vi "MRC Message Loop.vi"(8 "error in (no error)":errorcluster) -> (0 "error out":errorcluster)   [LabVIEW 2020, in "MRC Module.lvlib"]
doc: "Message loop for handling messages pertaining to the acquisition of data from the hardware."
uses:
  MRC Module.lvlib
  support/PCT FGV CMD.ctl
  Acquisition State.ctl
  MRC Configuration.ctl
  support/Message Queue/Message Cluster.ctl
  support/Message Queue/Enqueue Message (Single).vi
  support/Message Queue/Message Queue.lvlib
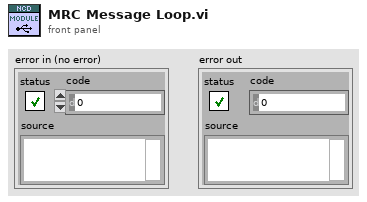
[diagram p1: front panel]
types:
  T1 = typedef "PCT FGV CMD.ctl" = enum16{"INIT", "GET", "SET"}
  T2 = typedef "Message Queue.lvlib/All Message Queues.ctl" = cluster{"UI":refnum<queue>, "Logging":refnum<queue>, "LOG":refnum<queue>, "ALARM":refnum<queue>, "Test":refnum<queue>, "Answer":refnum<queue>, "PLC":refnum<queue>, "DB":refnum<queue>, "Report":refnum<queue>, "OPC":refnum<queue>, "Procedure":refnum<queue>, "PalmSens":refnum<queue>, "SYS 7000 Reader":refnum<queue>, "SWITCH":refnum<queue>, "MOTOR":refnum<queue>, "MOTION":refnum<queue>, "HIDEN":refnum<queue>, "VALVE":refnum<queue>, "MFC":refnum<queue>, "PUMP IN":refnum<queue>, "PUMP OUT":refnum<queue>}
  T3 = typedef "PCT Data REFs.ctl" = cluster{"PLC AI Notifier":refnum<notifier>, "PS Data Queue":refnum<queue>, "BTN Queue":refnum<queue>, "PLC DI notifier":refnum<notifier>, "Timer notifier":refnum<notifier>, "DMM PS":refnum<notifier>, "DMM Gages":refnum<notifier>, "XYZ notifier":refnum<notifier>, "Test Notifier":refnum<notifier>, "Scanner notifier":refnum<notifier>, "OPC Notifier":refnum<notifier>, "HIDEN queue":refnum<queue>}
  T4 = typedef "MRC Module.lvlib/MRC Configuration.ctl" = cluster{"MFC Definition":cluster{"MFC Port":refnum<visa-resource-name>, "MFC Enable":bool, "Baud Rate":i32, "Interface type":enum32{"RS-485", "RS-232"}, "Address":i32}, "Set Point Options":cluster{"Setpoint Value":dbl, "Mass Flow EU 2":string, "Setpoint Source":string, "Valve Mode":string}, "Writer Queue":refnum<queue>, "Enable":bool, "Update Rate":u32, "MRC Chamber Enable":bool, "Selected Gas":string, "Address String":string}
  T5 = typedef "MRC Module.lvlib/Acquisition State.ctl" = enum16{"Idle", "Initialized"}
  T6 = typedef "Message Queue.lvlib/Message Cluster.ctl" = cluster{"Message":string, "Message Data":variant}
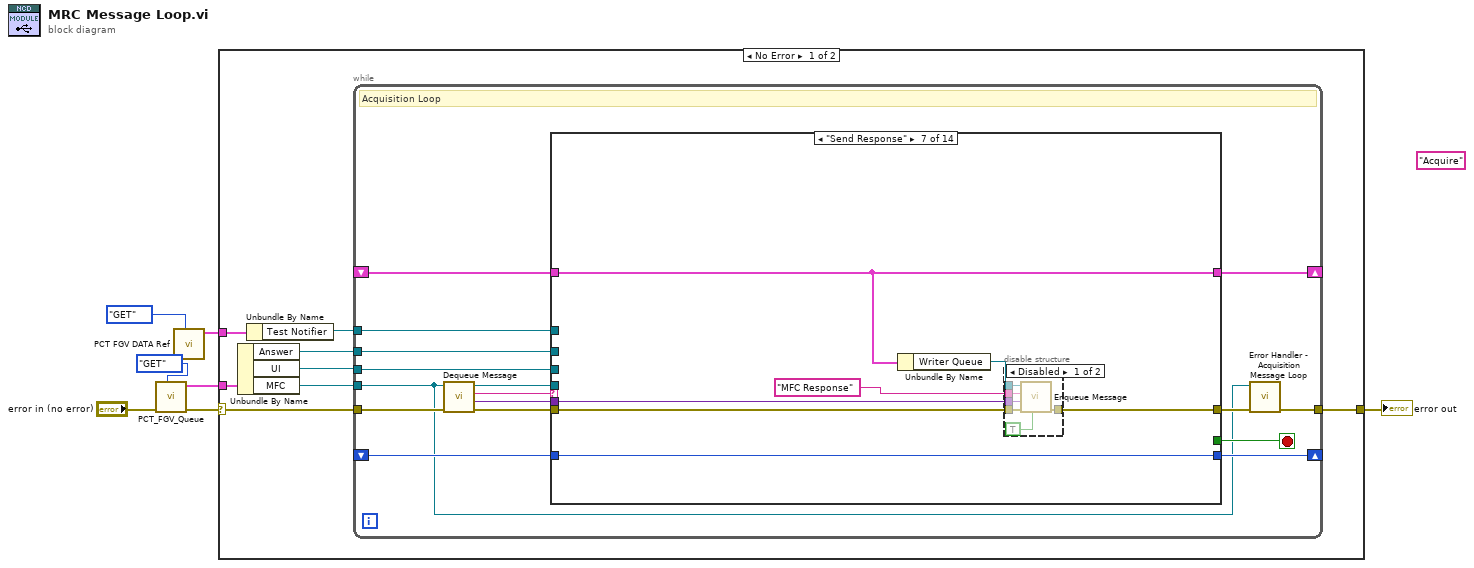
[diagram p0: block diagram]
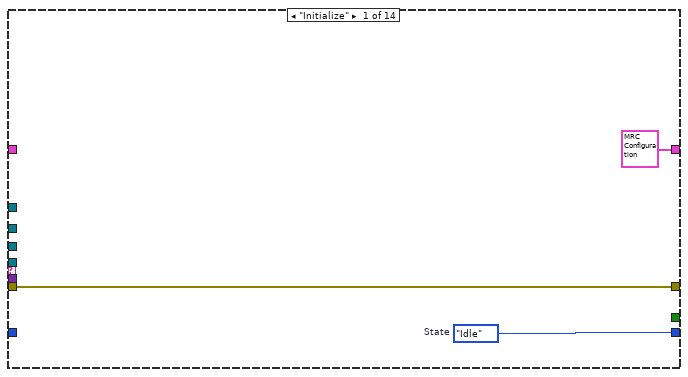
[diagram p2: hidden frame]
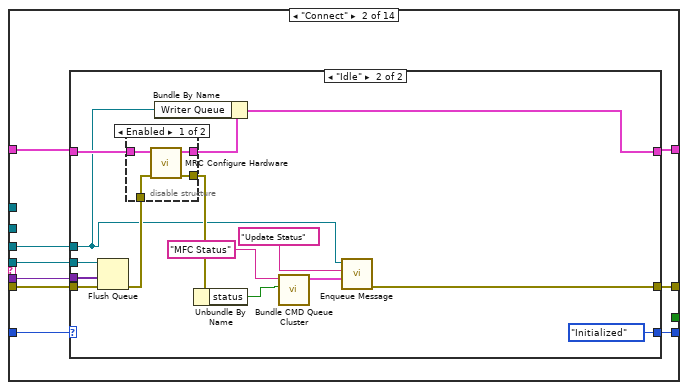
[diagram p3: hidden frame]
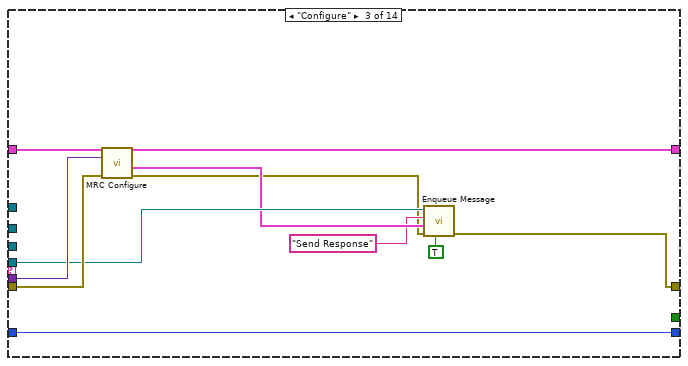
[diagram p6: hidden frame]
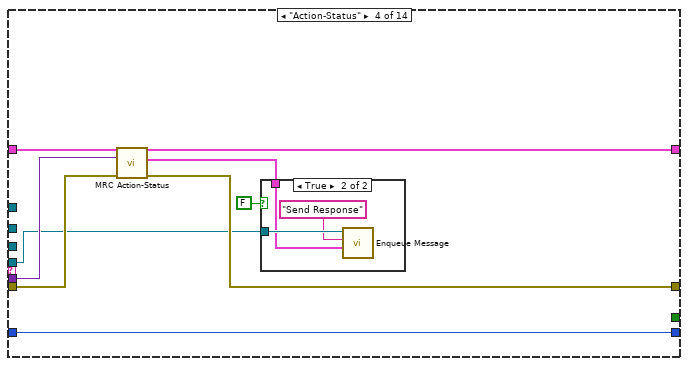
[diagram p7: hidden frame]
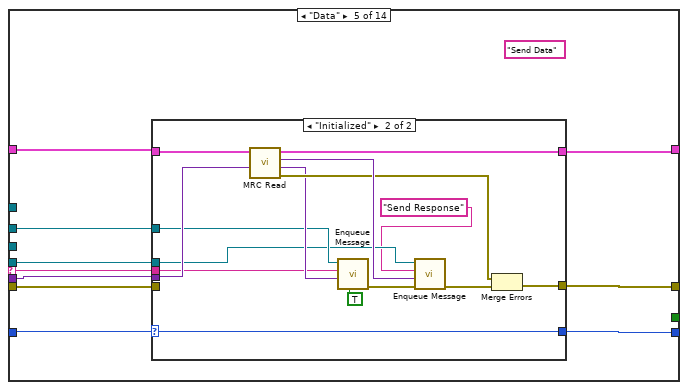
[diagram p9: hidden frame]
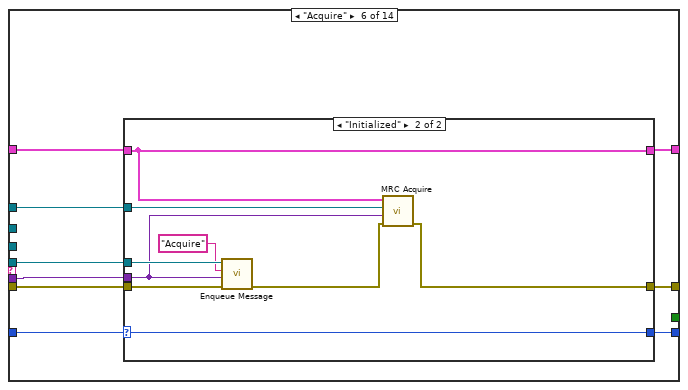
[diagram p11: hidden frame]
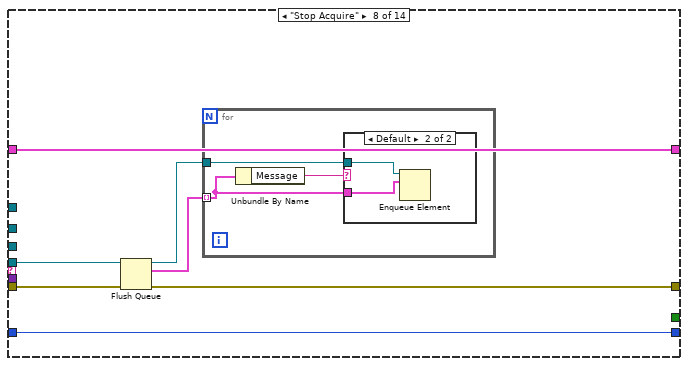
[diagram p14: hidden frame]
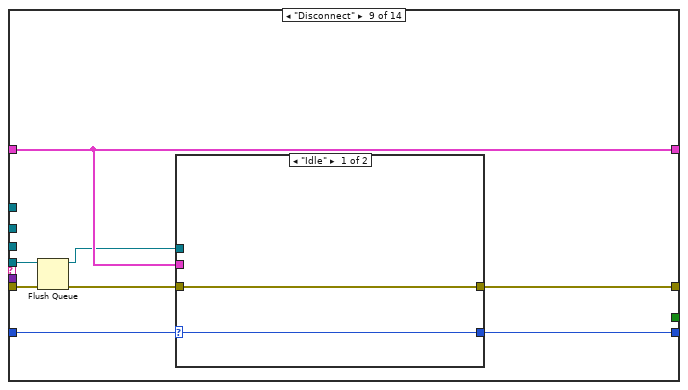
[diagram p16: hidden frame]
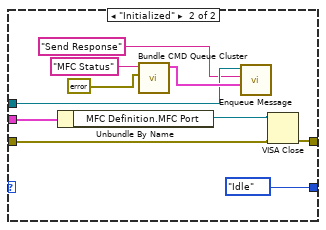
[diagram p17: hidden frame]
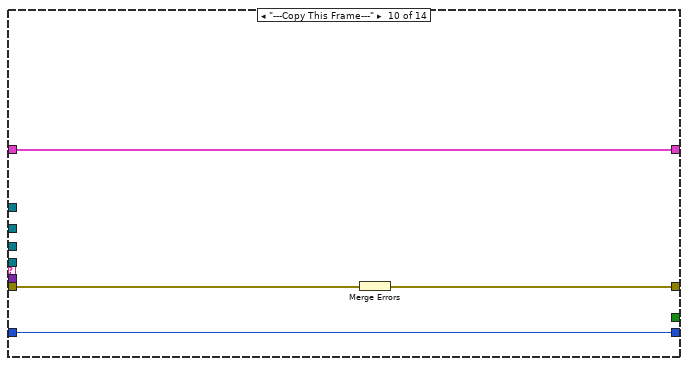
[diagram p18: hidden frame]
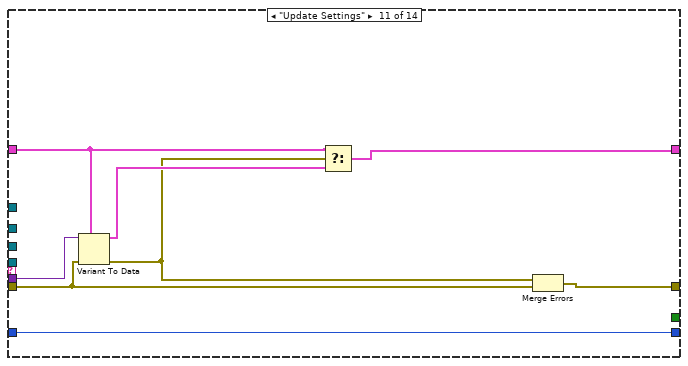
[diagram p19: hidden frame]
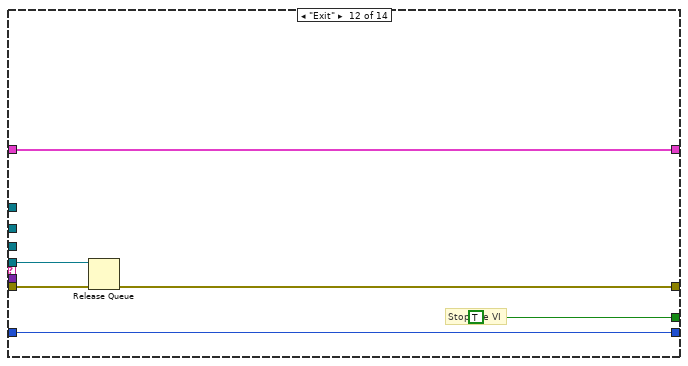
[diagram p20: hidden frame]
diagram:
  (unwired) "Acquire" ("Message")
  n1 = call "PCT_FGV_Queue.vi"("CMD"=PCT_FGV_CMD."GET", "error in (no error)"="error in (no error)") -> ("error out"=w2:errorcluster, "Message Queues out"=w1:T2)  [unwired: 8 in]
  n2 = call "PCT FGV DATA Ref.vi"("CMD"=PCT_FGV_CMD."GET") -> ("Data REF"=w5:T3)  [unwired: 9 in, 1 out]
  n3 = case shown="No Error" w2 {
    selector: w2 -> [w12 w219]
    tunnel: w1 -> [w15 _]
    tunnel: [w13 w219] -> w7
    tunnel: w5 -> [w10 _]
    frame No Error {
      n4 = Unbundle By Name(w15) -> ("Answer"=w8:refnum<queue>, "UI"=w11:refnum<queue>, "MFC"=w14:refnum<queue>)
      n5 = Unbundle By Name(w10) -> ("Test Notifier"=w9:refnum<notifier>)
      n6 = while {
        tunnel: w14 -> [w17]
        shift-right: [w30] -> _
        shift-left: _ -> [w31]
        tunnel: w11 -> [w21]
        shift-right: [w24] -> _
        shift-left: _ -> [w25]
        tunnel: w9 -> [w18]
        tunnel: w8 -> [w16]
        tunnel: w12 -> [w28]
        tunnel: [w19] -> w13
        stop <- w29 stop-if-true
        # "Acquisition Loop"
        n7 = call "Dequeue Message.vi"("error in (no error)"=w28, "Message Queue"=w17) -> ("error out"=w27:errorcluster, "Message Data"=w26:variant, "Message"=w22:string, "dup Message Queue"=w23:refnum<queue>)  [unwired: 6 in]
        n8 = case "Message Cases" shown="\"Send Response\"" w22 {
          selector: w22 -> [_ _ _ _ w91 _ _ _ _ _ _ _ _ _]
          tunnel: w23 -> [_ w40 w72 w78 w98 w125 _ w154 w164 _ _ w195 _ _]
          tunnel: w27 -> [w34 w41 w74 w82 w94 w119 w141 w155 w169 w186 w191 w197 w209 _]
          tunnel: [w34 w43 w67 w81 w99 w126 w140 w155 w170 w184 w194 w196 w210 errorcluster {"status"=FALSE, "code"=0, "source"=""} ("error out")] -> w20
          tunnel: w31 -> [_ w42 w75 w83 w93 w123 w144 w156 w168 w185 w187 w198 w213 w218]
          tunnel: [T4 {"MFC Definition"={"MFC Port"="", "MFC Enable"=TRUE, "Baud Rate"=0, "Interface type"=enum."RS-485", "Address"=0}, "Set Point Options"={"Setpoint Value"=0.0, "Mass Flow EU 2"="", "Setpoint Source"="", "Valve Mode"=""}, "Writer Queue"=refnum, "Enable"=FALSE, "Update Rate"=0, "MRC Chamber Enable"=FALSE, "Selected Gas"="", "Address String"=""} ("Data Cluster") w39 w73 w84 w97 w124 w144 w156 w168 w185 w188 w198 w213 w218] -> w30
          tunnel: [_ _ _ _ _ _ _ _ _ _ _ TRUE _ _] -> w29
          tunnel: w26 -> [_ w35 w76 w85 w95 w120 w139 _ _ _ w190 _ w208 _]
          tunnel: w21 -> [_ w36 _ _ _ _ _ _ _ _ _ _ w205 _]
          tunnel: w25 -> [_ w37 w77 w86 w92 w121 w145 w157 w167 w183 w193 w199 _ w217]
          tunnel: [w33 w38 w77 w86 w96 w122 w145 w157 w166 w183 w193 w199 Acquisition_State."Idle" ("State") w217] -> w24
          tunnel: w18 -> [_ _ _ _ _ w118 _ _ _ _ _ _ _ _]
          tunnel: w16 -> [_ _ _ _ w90 _ _ _ _ _ _ _ w204 _]
          frame "Initialize" {
            w33 = Acquisition_State."Idle"  # State
            # "Initialize  - Initialize is currently a no-op.  The hardware initialization takes place in the 'Start' message."
          }
          frame "Connect" {
            # "Start - Configure and start the acquisition."
            n9 = case shown="\"Idle\"" w37 {
              selector: w37 -> [w44 _]
              tunnel: [w45 w55] -> w43
              tunnel: w42 -> [w46 w60]
              tunnel: w41 -> [w45 w52]
              tunnel: w40 -> [_ w59]
              tunnel: [w46 w53] -> w39
              tunnel: [w44 Acquisition_State."Initialized" ("State")] -> w38
              tunnel: w36 -> [_ w48]
              tunnel: w35 -> [_ _]
              frame "Initialized" {
                # "The system is already acquiring. Ignore the \"Start\" message."
              }
              frame "Idle" {
                # "If the system is idle, start the acquisition."
                n10 = Flush Queue(queue=w59, error in (no error)=w52) -> (error out=w51:errorcluster)  [unwired: 2 out]
                n11 = disable-structure shown="Enabled" {
                  disable-tunnel: w60 -> [w64 w65]
                  disable-tunnel: [w63 w65] -> w54
                  disable-tunnel: w51 -> [w62 w66]
                  disable-tunnel: [w61 w66] -> w50
                  frame Enabled {
                    n12 = call "MRC Configure Hardware.vi"("error in (no error)"=w62, "Hardware Resources in"=w64) -> ("error out"=w61:errorcluster, "Hardware Resources out"=w63:T4)  [unwired: 8 in]
                  }
                  frame Disabled {
                  }
                }
                n13 = Bundle By Name(cluster=w54, "Writer Queue"=w48) -> (w53:T4)
                n14 = Unbundle By Name(w50) -> ("status"=w47:bool)
                n15 = call "Bundle CMD Queue Cluster.vi"("Message Data"=w47, "Message"="MFC Status" ("Type CMD")) -> ("Message Cluster"=w57:T6)  [unwired: 9 in]
                n16 = call-poly "Enqueue Message.vi"("Message Data"=w57, "Message"="Update Status", "Message Queue"=w48) -> ("error out"=w55:errorcluster)  [unwired: 7 in, 1 out]
              }
            }
          }
          frame "Configure" {
            # "Start - Configure and start the acquisition."
            n17 = call "MRC Configure.vi"("error in (no error)"=w74, "Message Data"=w76, "Data Cluster"=w75) -> ("error out"=w68:errorcluster, "Message"=w71:T6, "Data Cluster out"=w73:T4)  [unwired: 5 in, 1 out]
            n18 = call-poly "Enqueue Message.vi"("Priority Message? (F)"=TRUE, "error in (no error)"=w68, "Message Data"=w71, "Message"="Send Response", "Message Queue"=w72) -> ("error out"=w67:errorcluster)  [unwired: 5 in, 1 out]
          }
          frame "Action-Status" {
            # "Start - Configure and start the acquisition."
            n19 = call "MRC Action-Status.vi"("error in (no error)"=w82, "Message Data"=w85, "Data Cluster"=w83) -> ("error out"=w81:errorcluster, "Message"=w79:T6, "Data Cluster out"=w84:T4)  [unwired: 6 in]
            n20 = case shown="True" FALSE {
              tunnel: w78 -> [_ w89]
              tunnel: w79 -> [_ w87]
              frame False {
              }
              frame True {
                n21 = call-poly "Enqueue Message.vi"("Message Data"=w87, "Message"="Send Response", "Message Queue"=w89) -> ()  [unwired: 7 in, 2 out]
              }
            }
          }
          frame "Data" {
            (unwired) "Send Data" ("Message")
            # "Acquire - Acquire data from the hardware. Since this is a continuous acquisition, this message will always message itself to run again."
            n22 = case shown="\"Initialized\"" w92 {
              selector: w92 -> [w100 w116]
              tunnel: [w101 w117] -> w99
              tunnel: w98 -> [_ w104]
              tunnel: w94 -> [w101 _]
              tunnel: [w102 w111] -> w97
              tunnel: w93 -> [w102 w112]
              tunnel: [w100 w116] -> w96
              tunnel: w95 -> [_ w107]
              tunnel: w91 -> [_ w106]
              tunnel: w90 -> [_ w105]
              frame "Idle" {
              }
              frame "Initialized" {
                # "Read  data"
                n23 = call "MRC Read.vi"("Message Data"=w107, "Data  in"=w112) -> ("error out"=w109:errorcluster, "Message Data Out"=w108:variant, "Error Message"=w110:variant, "Data out"=w111:T4)  [unwired: 6 in]
                n24 = call-poly "Enqueue Message.vi"("Priority Message? (F)"=TRUE, "Message Data"=w108, "Message"=w106, "Message Queue"=w105) -> ("error out"=w115:errorcluster)  [unwired: 6 in, 1 out]
                n25 = call-poly "Enqueue Message.vi"("error in (no error)"=w115, "Message Data"=w110, "Message"="Send Response", "Message Queue"=w104) -> ("error out"=w114:errorcluster)  [unwired: 6 in, 1 out]
                n26 = Merge Errors(w109, w114) -> (w117:errorcluster)
              }
            }
          }
          frame "Acquire" {
            # "Acquire - Acquire data from the hardware. Since this is a continuous acquisition, this message will always message itself to run again."
            n27 = case shown="\"Initialized\"" w121 {
              selector: w121 -> [w127 w136]
              tunnel: [w128 w130] -> w126
              tunnel: w125 -> [_ w138]
              tunnel: w119 -> [w128 w135]
              tunnel: [w129 w131] -> w124
              tunnel: w123 -> [w129 w131]
              tunnel: [w127 w136] -> w122
              tunnel: w120 -> [_ w133]
              tunnel: w118 -> [_ w134]
              frame "Idle" {
              }
              frame "Initialized" {
                # "Read  data"
                n28 = call-poly "Enqueue Message.vi"("error in (no error)"=w135, "Message Data"=w133, "Message"="Acquire", "Message Queue"=w138) -> ("error out"=w132:errorcluster)  [unwired: 6 in, 1 out]
                n29 = call "MRC Acquire.vi"("error in (no error)"=w132, "Message Data"=w133, "MRC notifier"=w134, "Hardware Resources in"=w131) -> ("error out"=w130:errorcluster)  [unwired: 6 in, 1 out]
              }
            }
          }
          frame "Send Response" {
            # "Acquire - Acquire data from the hardware. Since this is a continuous acquisition, this message will always message itself to run again."
            n30 = Unbundle By Name(w144) -> ("Writer Queue"=w143:refnum<queue>)
            n31 = disable-structure shown="Disabled" {
              disable-tunnel: w143 -> [w151 _]
              disable-tunnel: "MFC Response" ("Message") -> [w150 _]
              disable-tunnel: w141 -> [w149 _]
              disable-tunnel: [w148 _] -> w140
              disable-tunnel: w139 -> [w147 _]
              frame Disabled {
                n32 = call-poly "Enqueue Message.vi"("Priority Message? (F)"=TRUE, "error in (no error)"=w149, "Message Data"=w147, "Message"=w150, "Message Queue"=w151) -> ("error out"=w148:errorcluster)  [unwired: 5 in, 1 out]
              }
              frame Enabled {
              }
            }
          }
          frame "Stop Acquire" {
            # "Acquire - Acquire data from the hardware. Since this is a continuous acquisition, this message will always message itself to run again."
            n33 = Flush Queue(queue=w154) -> (queue out=w152:refnum<queue>, remaining elements=w153:T6[])  [unwired: 1 in, 1 out]
            n34 = for {
              tunnel: w153 -> [w159] mode=indexing
              tunnel: w152 -> [w158]
              n35 = Unbundle By Name(w159) -> ("Message"=w160:string)
              n36 = case shown="Default" w160 {
                tunnel: w159 -> [_ w162]
                tunnel: w158 -> [_ w161]
                frame "Acquire" {
                }
                frame Default {
                  n37 = Enqueue Element(queue=w161, element=w162) -> ()  [unwired: 2 in, 3 out]
                }
              }
            }
          }
          frame "Disconnect" {
            # "Stop - Stop the Acquisition."
            n38 = Flush Queue(queue=w164, error in (no error)=w169) -> (queue out=w163:refnum<queue>, error out=w165:errorcluster)  [unwired: 1 out]
            n39 = case shown="\"Idle\"" w167 {
              selector: w167 -> [w171 _]
              tunnel: w165 -> [w172 w174]
              tunnel: [w172 w173] -> w170
              tunnel: w168 -> [_ w176]
              tunnel: [w171 Acquisition_State."Idle" ("State")] -> w166
              tunnel: w163 -> [_ w178]
              frame "Idle" {
                # "The system is already idle. Ignore the \"Stop\" message."
              }
              frame "Initialized" {
                # "If the system is acquiring, stop the acquisition."
                n40 = Unbundle By Name(w176) -> ("MFC Definition.MFC Port"=w175:refnum<visa-resource-name>)
                n41 = call "Bundle CMD Queue Cluster.vi"("Message Data"=errorcluster {"status"=TRUE, "code"=0, "source"=""} ("error out"), "Message"="MFC Status" ("Type CMD")) -> ("Message Cluster"=w180:T6)  [unwired: 9 in]
                n42 = call-poly "Enqueue Message.vi"("Message Data"=w180, "Message"="Send Response", "Message Queue"=w178) -> ()  [unwired: 7 in, 2 out]
                n43 = VISA Close(VISA resource name=w175, error in (no error)=w174) -> (error out=w173:errorcluster)
              }
            }
          }
          frame "---Copy This Frame---" {
            # "Duplicate this frame when creating new messages.  Change this comment in the duplicated frame to describe this message."
            n44 = Merge Errors(w186) -> (w184:errorcluster)
          }
          frame "Update Settings" {
            # "New settings are available, update the current ones stored in the shift register with the settings sent as part of the message"
            n45 = Variant To Data(error in=w191, type=w187, Variant=w190) -> (data=w192:T4, error out=w189:errorcluster)
            n46 = Select(t=w187, s=w189, f=w192) -> (s? t:f=w188:T4)
            n47 = Merge Errors(w189, w191) -> (w194:errorcluster)
          }
          frame "Exit" {
            # "Stop the VI"
            # "Exit - Send the Exit message to the UI Message Handler."
            n48 = Release Queue(queue=w195, error in (no error)=w197) -> (error out=w196:errorcluster)  [unwired: 1 in, 2 out]
          }
          frame "Error" {
            w202 = "MFC MSG" ("Type CMD")
            n49 = Variant To Data(type=w209, Variant=w208) -> (data=w212:errorcluster)  [unwired: 1 in, 1 out]
            n50 = Unbundle By Name(w212) -> ("source"=w201:string, "code"=w211:i32)
            n51 = case shown="0, Default" w211 {
              tunnel: w201 -> [_ _ _ w215]
              frame 0, Default {
                n52 = Two Button Dialog(message="MFC Error") -> ()  [unwired: 2 in, 1 out]
              }
              frame 5102 {
              }
              frame 5100 {
              }
              frame -1073807339 {
                n53 = One Button Dialog(message=w215) -> ()  [unwired: 1 in, 1 out]
              }
            }
            n54 = call "Bundle CMD Queue Cluster.vi"("Message Data"=w201, "Message"=w202) -> ("Message Cluster"=w203:T6)  [unwired: 9 in]
            n55 = call-poly "Enqueue Message.vi"("Message Data"=w203, "Message"="MFC Response", "Message Queue"=w205) -> ()  [unwired: 7 in, 2 out]
            n56 = call-poly "Enqueue Message.vi"("Message Data"=w201, "Message"=w202, "Message Queue"=w204) -> ()  [unwired: 7 in, 2 out]
            n57 = call <vilib>:"Clear Errors.vi"("error in (no error)"=w209) -> ("error out"=w210:errorcluster)  [unwired: 5 in, 1 out]
          }
          frame Default {
            # "'Default' case only runs if there is a message that isn't defined in any of the other cases.  Output a programming error."
          }
        }
        n58 = call "Error Handler - Acquisition Message Loop.vi"("error in (no error)"=w20, "Message Queue"=w17) -> ("dup error in"=w19:errorcluster)  [unwired: 8 in, 1 out]
      }
    }
    frame Error {
    }
  }
  "error out" <- w7
